vi "SRV_Motor Button - Is Any Active.vi"(7 "Motor Control Button":T1 {"Release Cmds"."Motor Control Commands Array"."Value" format="%02x"; "Release Cmds"."Motor Control Commands Array"."Register" format="%02x"; "Release Cmds"."Motor Control Commands Array"."I2C Address" format="%02x"; "Press Cmds"."Motor Control Commands Array"."Value" format="%02x"; "Press Cmds"."Motor Control Commands Array"."Register" format="%02x"; "Press Cmds"."Motor Control Commands Array"."I2C Address" format="%02x"}) -> (8 "Motor Control Button dup":T1 {"Release Cmds"."Motor Control Commands Array"."Value" format="%02x"; "Release Cmds"."Motor Control Commands Array"."Register" format="%02x"; "Release Cmds"."Motor Control Commands Array"."I2C Address" format="%02x"; "Press Cmds"."Motor Control Commands Array"."Value" format="%02x"; "Press Cmds"."Motor Control Commands Array"."Register" format="%02x"; "Press Cmds"."Motor Control Commands Array"."I2C Address" format="%02x"}, 10 "Any Active?":bool)   [LabVIEW 2014]
uses:
  Motors Config/SRV_Motor Control Button Config.ctl
  Motors Config/SRV_Motor Legos-Servo.ctl
  Motors Config/SRV_Motor Control Commands Cluster.ctl
  Motors Config/SRV_Motor Control Command Config.ctl
  Motors Config/SRV_Motor Control Button Icons_FALSE.ctl
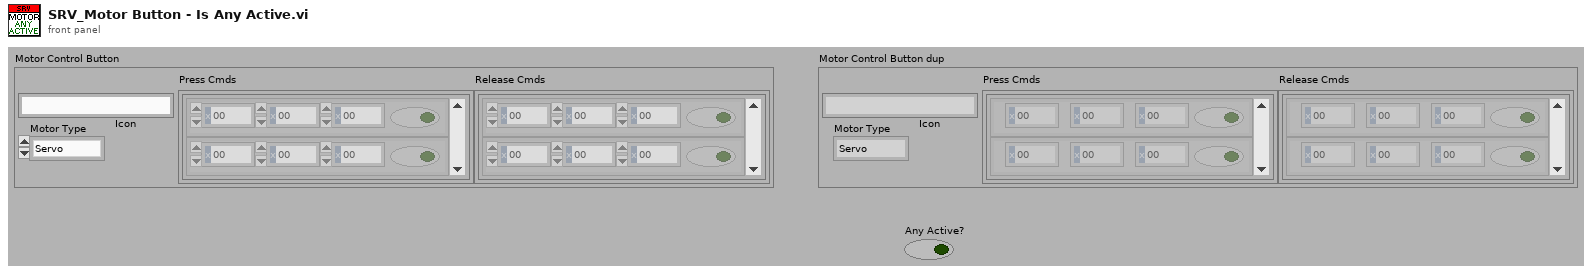
[diagram p1: front panel]
types:
  T1 = typedef "SRV_Motor Control Button Config.ctl" = cluster{"Button Name":string, "Button Label":string, "Motor Type":T2, "Press Cmds":T3, "Release Cmds":T3, "Icon":T5}
  T2 = typedef "SRV_Motor Legos-Servo.ctl" = enum16{"Servo", "Legos", "Shared Var"}
  T3 = typedef "SRV_Motor Control Commands Cluster.ctl" = cluster{"Motor Control Commands Array":T4[]}
  T4 = typedef "SRV_Motor Control Command Config.ctl" = cluster{"I2C Address":u8, "Register":u8, "Value":u8, "Active":bool}
  T5 = typedef "SRV_Motor Control Button Icons_FALSE.ctl" = u16
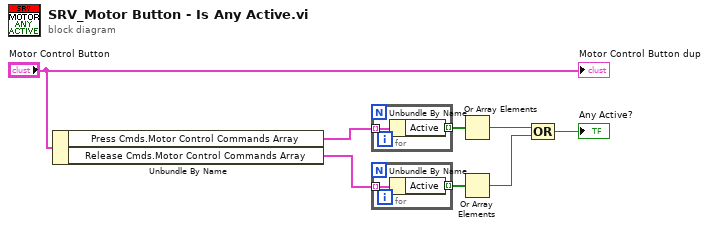
[diagram p0: block diagram]
diagram:
  n1 = Unbundle By Name("Motor Control Button") -> ("Press Cmds.Motor Control Commands Array"=w4:T4[], "Release Cmds.Motor Control Commands Array"=w8:T4[])
  n2 = for {
    tunnel: w4 -> [w10] mode=indexing
    tunnel: [w9] -> w3 mode=indexing
    n3 = Unbundle By Name(w10) -> ("Active"=w9:bool)
  }
  n4 = for {
    tunnel: w8 -> [w12] mode=indexing
    tunnel: [w11] -> w6 mode=indexing
    n5 = Unbundle By Name(w12) -> ("Active"=w11:bool)
  }
  n6 = Or Array Elements(Boolean array=w3) -> (logical OR=w5:bool)
  n7 = Or Array Elements(Boolean array=w6) -> (logical OR=w7:bool)
  n8 = Compound Arithmetic op=OR(w5, w7) -> (→"Any Active?":bool)
  "Motor Control Button dup" <- "Motor Control Button"
